vi "GlueRepeatedLinePattern-TeachMode.vi"(0 "Calibration Directory":path, 1 "Module Number":i32=7, 2 "Stereo Angle [mrad]":dbl=-26.0 format="%#_13g", 3 "Dry Run":bool, 4 "Controller In":refnum<k24>) -> ()   [LabVIEW 2016]
uses:
  <vilib>/LabVIEW Interface for Arduino/Type Defs/Arduino Resource.ctl
  <vilib>/LabVIEW Interface for Arduino/Type Defs/Board Type.ctl
  C:/Users/Aerotech/Documents/BNLStaveAssembly-blueprint/Bin/Aerotech.A3200.dll
  BNLStaveAssembly-blueprint/Bin/Aerotech.A3200.dll
  <vilib>/LabVIEW Interface for Arduino/Type Defs/Pin Mode.ctl
  <vilib>/Utility/file.llb/Read Delimited Spreadsheet (DBL).vi
  <vilib>/LabVIEW Interface for Arduino/LabVIEW Interface for Arduino.lvlib
panel:
  out "N Lines":i32
  out "Lines Glued":i32
  out "Elapsed Time [s]":dbl format="%.2g"
  out "Finished":bool
  in  "Abort stage":bool
  in  "Pattern Indicator":enum32{"Glue Pattern"}(tab)
  out "Relative Line\nSeparations [mm]":dbl[][](array[numeric])=[[18.5, 7.25], [2.5, 3.5], [-3.5, 5.0], [2.5, 3.15], [2.5, 3.15], [2.5, 3.15], [2.5, 3.15], [2.5, 3.15], [2.5, 3.15], [2.5, 3.15], [2.5, 3.15], [2.5, 3.15], [2.5, 3.15], [2.5, 3.15], [3.75, 5.0], [2.5, 3.5]] format="%#_13g"
  out "Line Lengths [mm]":dbl[](array[numeric])=[65.0, 65.0, 73.5, 73.5, 73.5, 73.5, 73.5, 73.5, 73.5, 73.5, 73.5, 73.5, 73.5, 73.5, 65.0, 65.0] format="%#_13g"
  out "Line Speeds [mm/s]":dbl[][](array[numeric])=[[5.0, 5.0, 75.0, 75.0, 75.0, 75.0], [5.0, 5.0, 0.0, 0.0, 0.0, 0.0], [7.5, 7.5, 0.0, 0.0, 0.0, 0.0], [7.5, 7.5, 0.0, 0.0, 0.0, 0.0], [7.5, 7.5, 0.0, 0.0, 0.0, 0.0], [7.5, 7.5, 0.0, 0.0, 0.0, 0.0], [7.5, 7.5, 0.0, 0.0, 0.0, 0.0], [7.5, 7.5, 0.0, 0.0, 0.0, 0.0], [7.5, 7.5, 0.0, 0.0, 0.0, 0.0], [7.5, 7.5, 0.0, 0.0, 0.0, 0.0], [7.5, 7.5, 0.0, 0.0, 0.0, 0.0], [7.5, 7.5, 0.0, 0.0, 0.0, 0.0], [7.5, 7.5, 0.0, 0.0, 0.0, 0.0], [7.5, 7.5, 0.0, 0.0, 0.0, 0.0], [5.0, 5.0, 0.0, 0.0, 0.0, 0.0], [5.0, 5.0, 0.0, 0.0, 0.0, 0.0]] format="%#_13g"
  in  "Outputs Tab":enum32{"Running Positions"}(tab)
  out "Running Positions [mm]":dbl[][](array[numeric])
  in  "Times [s]":dbl[](array[numeric])
  out "Running Times [s]":dbl[](array[numeric])
  in  "Inputs Tab":T1(tab)
  out "Virtual Stave Map":path
  out "Stave Angle [rad]":dbl format="%#_13g"
  out "Total Angle [rad]":dbl
  in  "Pause Before Line [ms]":dbl=500.0 format="%#_13g"
  out "Arduino Resource":T2={"VISA resource"="GlueCTRL", "Board Type"=enum."Uno", "Connection Type"=enum."USB / Serial", "Bytes Per Packet (15)"=15}
  in  "Digital I/O Pin":u8=7
  in  "Default Axis Speeds":T4={"X [mm/s]"=25.0, "Y [mm/s]"=25.0, "Z [mm/s]"=25.0}
  in  "Pause After Line [ms]":dbl=1000.0 format="%#_13g"
  in  "Fine Axis Speeds [mm/s]":T4={"X [mm/s]"=15.0, "Y [mm/s]"=15.0, "Z [mm/s]"=15.0}
  in  "Camera to Dispenser Shift [mm]":dbl[](array[numeric])=[100.0, 0.0, -10.0]
  in  "Glue Pattern .csv File":path=path "C:/Users/Aerotech/Documents/BNL_ThermomechanicalStave/SchillaciGlue/GluePatterns/TimingAccuracy.txt"
  in  "Axial":bool
  in  "Positions [mm]":dbl[][](array[numeric])
  in  "Terminate":bool
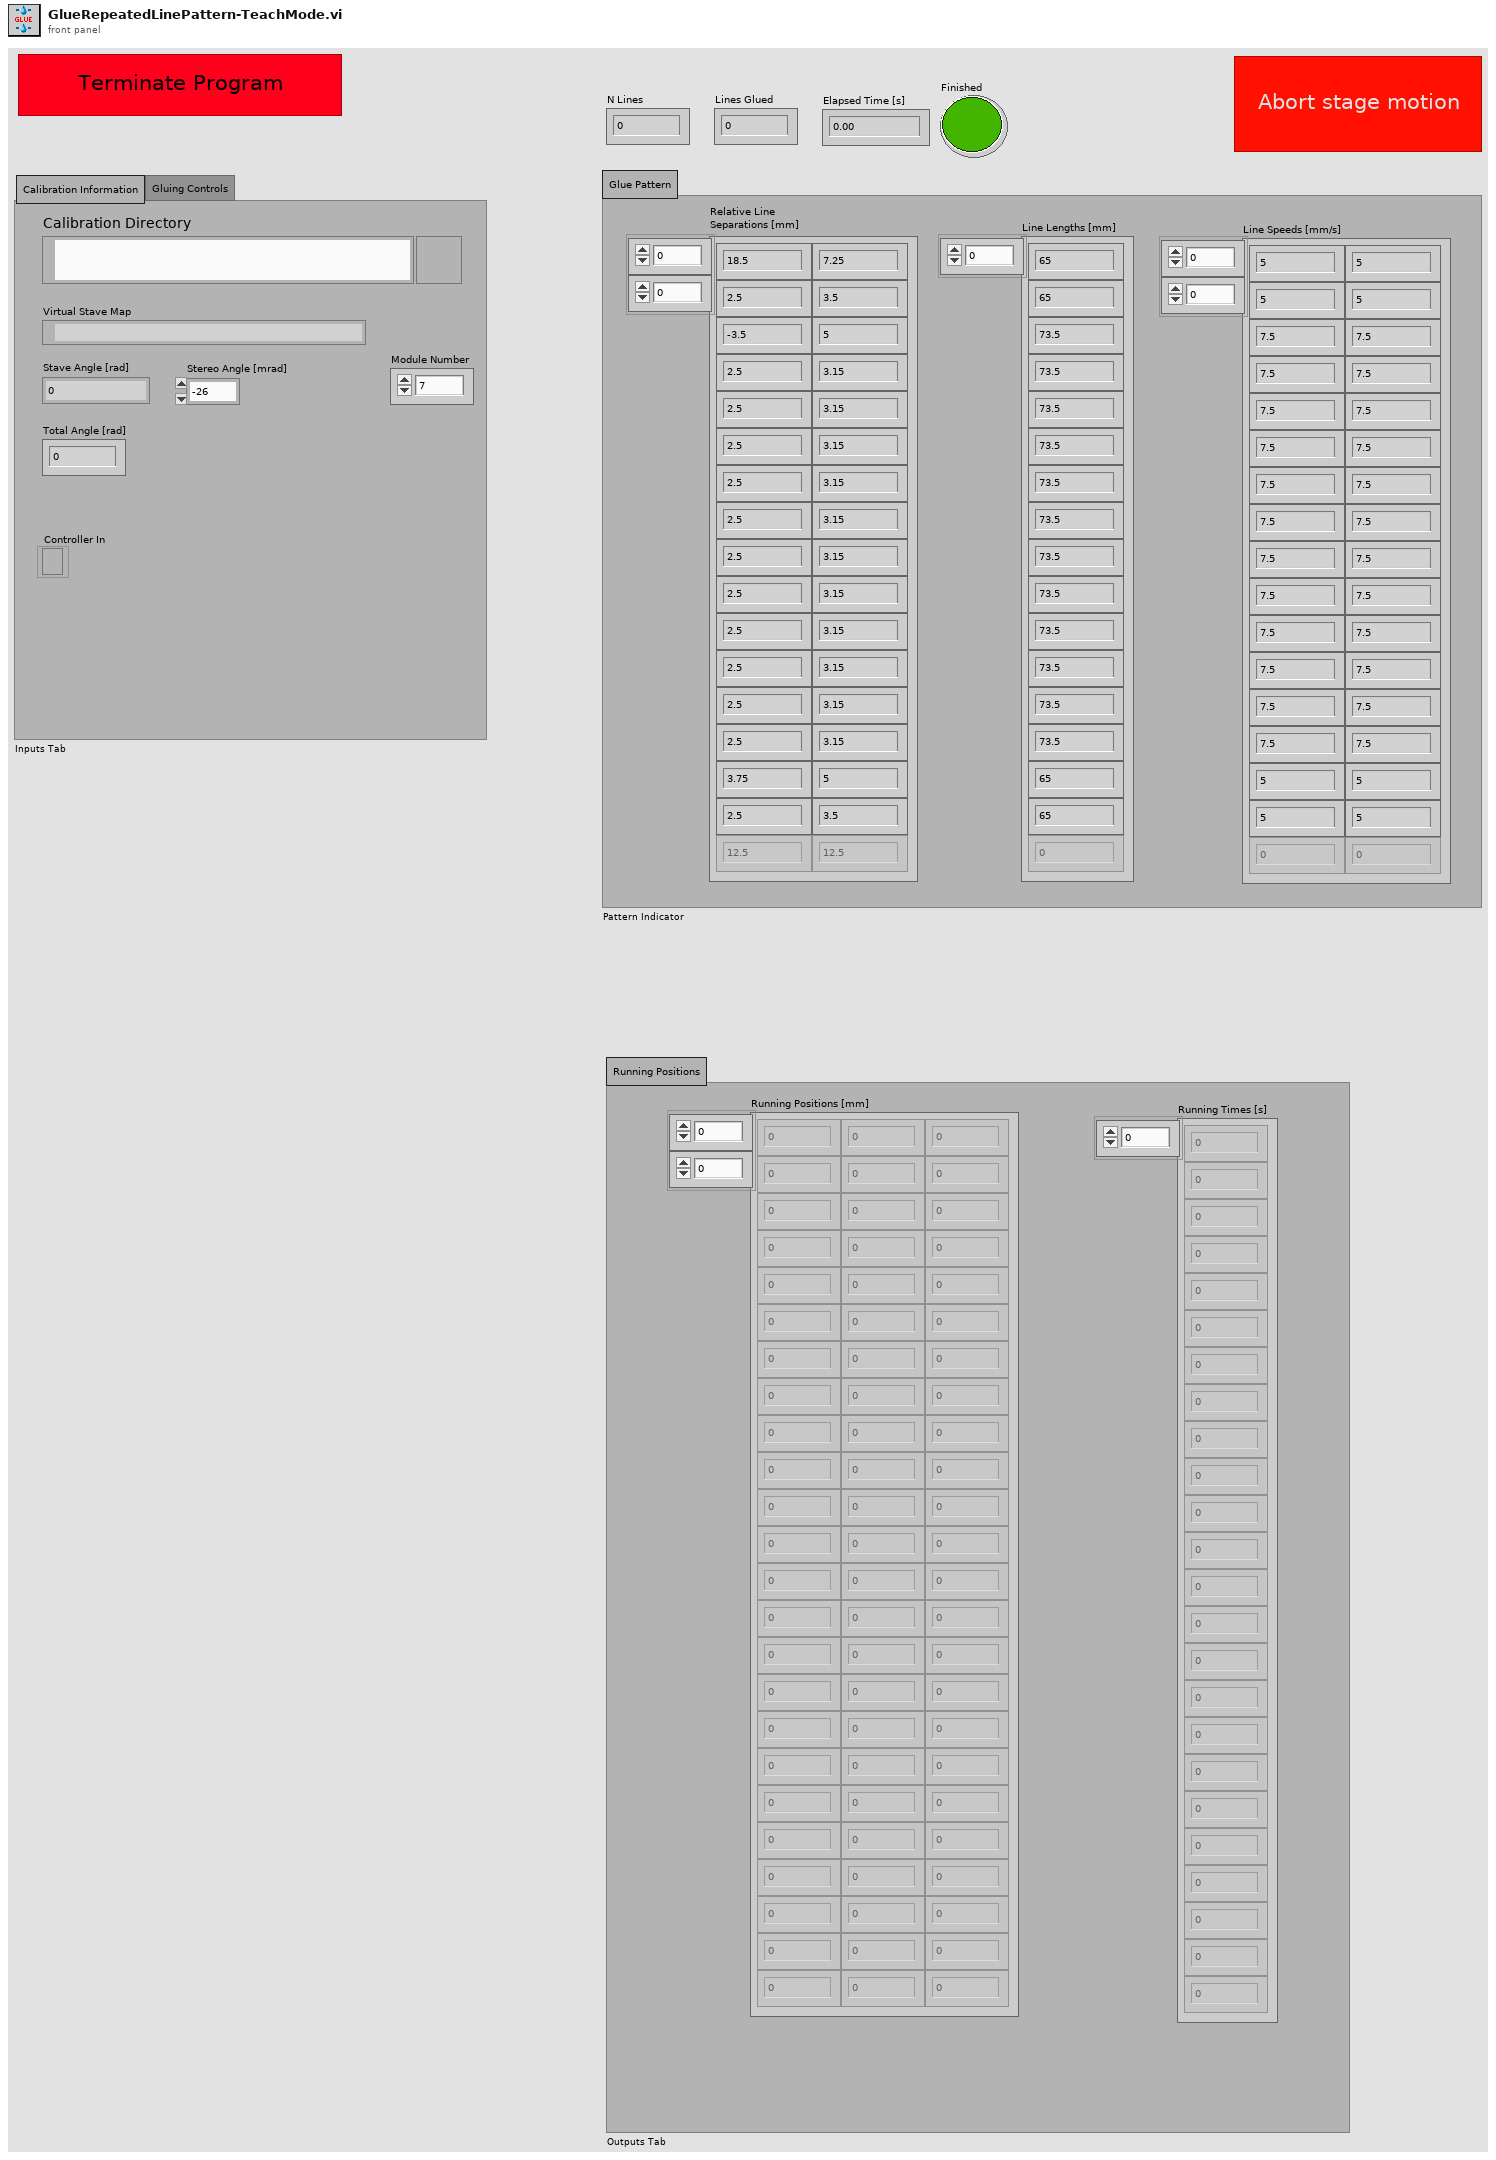
[diagram p1: front panel]
types:
  T1 = enum32{"Calibration Information", "Gluing Controls"}
  T2 = typedef "LabVIEW Interface for Arduino.lvlib/Arduino Resource.ctl" = cluster{"VISA resource":refnum<visa-resource-name>, "Board Type":T3, "Connection Type":enum8{"USB / Serial"}, "Bytes Per Packet (15)":u8}
  T3 = typedef "LabVIEW Interface for Arduino.lvlib/Board Type.ctl" = enum16{"Uno", "Dimuelanove w/Atmega 328", "Mega 2560"}
  T4 = cluster{"X [mm/s]":dbl, "Y [mm/s]":dbl, "Z [mm/s]":dbl}
  T5 = typedef "LabVIEW Interface for Arduino.lvlib/Pin Mode.ctl" = enum8{"Input", "Output"}
  T6 = cluster{"Final X":dbl, "Final Y":dbl, "Final Z":dbl}
  T7 = cluster{"Numeric":dbl, "Numeric":dbl, "Z [mm/s]":dbl}
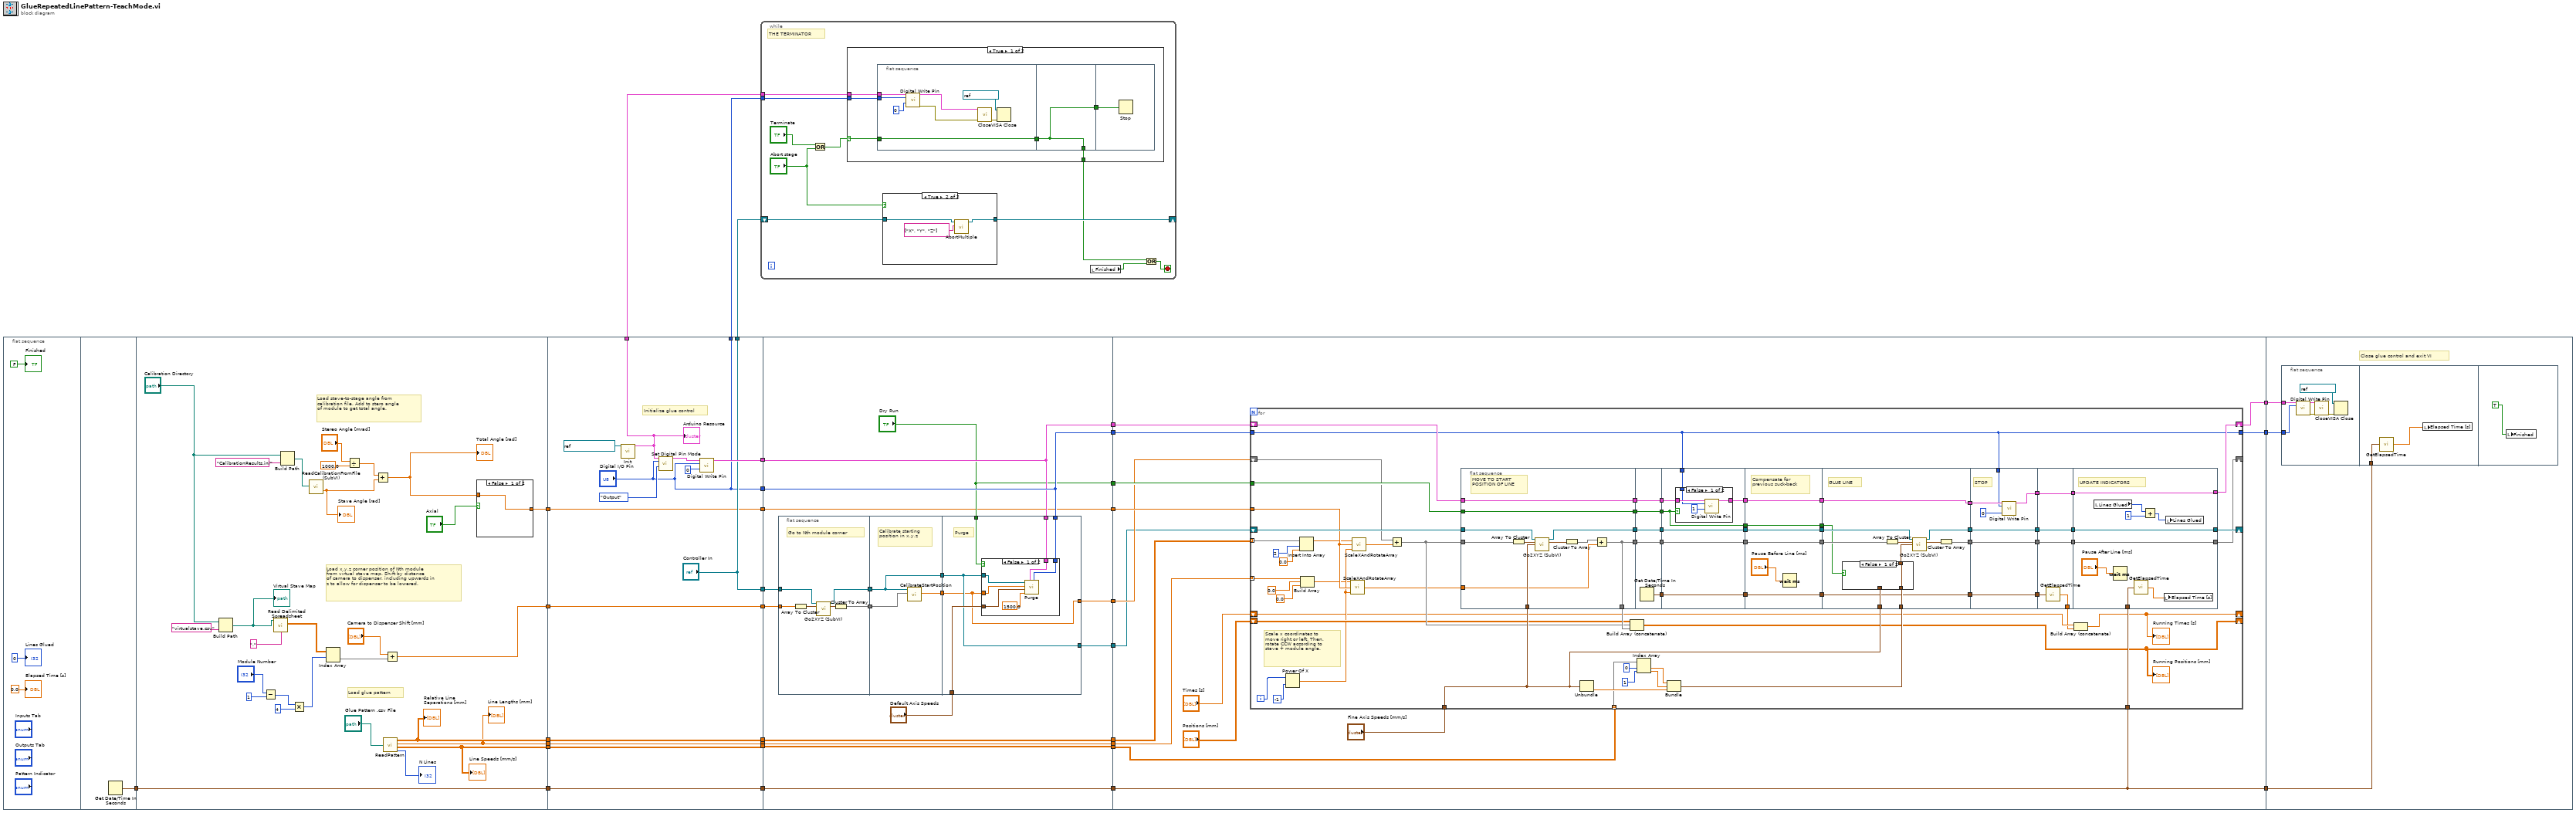
[diagram p0: block diagram]
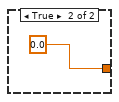
[diagram p2: hidden frame]
diagram:
  n1 = flat-sequence {
    tunnel: [w36] -> w16
    tunnel: [w49] -> w32
    tunnel: w16 -> [w46]
    tunnel: [w46] -> w15
    tunnel: [w38] -> w11
    tunnel: [w42] -> w5
    tunnel: [w41] -> w4
    tunnel: [w40] -> w2
    tunnel: w32 -> [w76]
    tunnel: [w76] -> w31
    tunnel: ["Controller In"] -> w30
    tunnel: [w75] -> w29
    tunnel: ["Digital I/O Pin"] -> w28
    tunnel: [w74] -> w22
    tunnel: ["Controller In"] -> w21
    tunnel: [w71] -> w18
    tunnel: w15 -> [w72]
    tunnel: [w72] -> w14
    tunnel: w11 -> [w71]
    tunnel: ["Digital I/O Pin"] -> w10
    tunnel: [w69] -> w6
    tunnel: w5 -> [w69]
    tunnel: w4 -> [w68]
    tunnel: [w68] -> w3
    tunnel: w2 -> [w67]
    tunnel: [w67] -> w1
    tunnel: w31 -> [w92]
    tunnel: w30 -> [w91]
    tunnel: w29 -> [w89]
    tunnel: w28 -> [w90]
    tunnel: [w90] -> w25
    tunnel: [w89] -> w24
    tunnel: [w88] -> w23
    tunnel: ["Dry Run"] -> w20
    tunnel: [w86] -> w19
    tunnel: w18 -> [w86]
    tunnel: [w85] -> w17
    tunnel: w14 -> [w84]
    tunnel: [w84] -> w13
    tunnel: [w83] -> w9
    tunnel: [w82] -> w8
    tunnel: [w81] -> w7
    tunnel: w6 -> [w83]
    tunnel: w3 -> [w82]
    tunnel: w1 -> [w81]
    tunnel: [w120] -> w27
    tunnel: [w131] -> w26
    tunnel: w25 -> [w130]
    tunnel: w24 -> [w129]
    tunnel: w23 -> [w125]
    tunnel: w20 -> [w128]
    tunnel: w19 -> [w127]
    tunnel: w17 -> [w126]
    tunnel: w13 -> [w124]
    tunnel: [w124] -> w12
    tunnel: w9 -> [w123]
    tunnel: w8 -> [w121]
    tunnel: w7 -> [w122]
    tunnel: w27 -> [w273]
    tunnel: w26 -> [w272]
    tunnel: w12 -> [w271]
    frame #0 {
      "Finished" <- FALSE ("Finished")
      "Elapsed Time [s]" <- 0.0 ("Elapsed Time [s]")
      "Lines Glued" <- 0 ("N Lines")
    }
    frame #1 {
      n2 = Get Date/Time In Seconds() -> (seconds since 1Jan1904=w36:timestamp)
    }
    frame #2 {
      # "Load glue pattern"
      # "Load x,y,z corner position of Nth module\nfrom virtual stave map. Shift by distance\nof camera to dispenser, including upwards in\nz to allow for dispenser to be lowered."
      # "Load stave-to-stage angle from\ncalibration file. Add to stero angle\nof module to get total angle."
      n3 = Build Path(base path="Calibration Directory", name or relative path="virtualstave.csv") -> (appended path=w58:path)
      "Virtual Stave Map" <- w58
      n4 = Subtract(x="Module Number", y=1) -> (x-y=w54:i32)
      n5 = call-poly <vilib>:"Read Delimited Spreadsheet.vi"("file path (dialog if empty)"=w58, "delimiter (\\t)"="," ("delimiter (\\t)")) -> ("all rows"=w50:dbl[][])  [unwired: 8 in, 5 out]
      n6 = Build Path(base path="Calibration Directory", name or relative path="CalibrationResults.ini") -> (appended path=w60:path)
      n7 = Multiply(x=w54, y=4) -> (x*y=w47:i32)
      n8 = call "ReadCalibrationFromFile (SubVI).vi"("Calibration file path"=w60) -> ("Angle"=w51:dbl)  [unwired: 12 in, 6 out]
      "Stave Angle [rad]" <- w51
      n9 = Index Array(array=w50, index (row)=w47) -> (element=w48:dbl[])  [unwired: 1 in]
      n10 = Divide(x="Stereo Angle [mrad]", y=1000.0) -> (x/y=w52:dbl)
      n11 = Add(x=w52, y=w51) -> (x+y=w37:dbl)
      "Total Angle [rad]" <- w37
      n12 = call "ReadPattern.vi"("file path (dialog if empty)"="Glue Pattern .csv File") -> ("Relative Line\nSeparations [mm]"=w42:dbl[][], "Line Lengths [mm]"=w41:dbl[], "Line Speeds [mm/s]"=w40:dbl[][], "N Lines"=→"N Lines":i32)
      "Relative Line\nSeparations [mm]" <- w42
      "Line Lengths [mm]" <- w41
      "Line Speeds [mm/s]" <- w40
      n13 = Add(x="Camera to Dispenser Shift [mm]", y=w48) -> (x+y=w49:dbl[])
      n14 = case shown="False" "Axial" {
        tunnel: [w65 0.0] -> w38
        tunnel: w37 -> [w65 _]
        frame False {
        }
        frame True {
        }
      }
    }
    frame #3 {
      # "Initialize glue control"
      n15 = call <vilib>:"Init.vi"("VISA resource"=refnum<visa-resource-name> "GlueCTRL") -> ("Arduino Resource"=w74:T2)  [unwired: 17 in, 1 out]
      "Arduino Resource" <- w74
      n16 = call <vilib>:"Set Digital Pin Mode.vi"("Arduino Resource"=w74, "Digital I/O Pin"="Digital I/O Pin", "Pin Mode (Input)"=Pin_Mode."Output") -> ("Arduino Resource"=w78:T2)  [unwired: 11 in, 1 out]
      n17 = call <vilib>:"Digital Write Pin.vi"("Arduino Resource"=w78, "Digital I/O Pin (0)"="Digital I/O Pin", "Value (0)"=u8 0) -> ("Arduino Resource"=w75:T2)  [unwired: 11 in, 1 out]
    }
    frame #4 {
      n18 = flat-sequence {
        tunnel: w91 -> [w101]
        tunnel: [w100] -> w97
        tunnel: w92 -> [w99]
        tunnel: [w98] -> w96
        tunnel: w97 -> [w105]
        tunnel: w96 -> [w106]
        tunnel: [w105] -> w95
        tunnel: [w104] -> w94
        tunnel: w95 -> [w109]
        tunnel: w94 -> [w107]
        tunnel: "Default Axis Speeds" -> [w112]
        tunnel: w90 -> [w111]
        tunnel: w89 -> [w110]
        tunnel: [w109] -> w88
        tunnel: "Dry Run" -> [w108]
        tunnel: [w107] -> w85
        frame #0 {
          # "Go to Nth module corner"
          n19 = Array To Cluster(array=w99) -> (cluster=w103:cluster{"[0]":dbl, "[1]":dbl, "[2]":dbl})
          n20 = call "Go2XYZ (SubVI).vi"(".NET Refnum in"=w101, "Go to Coordinates"=w103) -> (".NET Refnum out"=w100:refnum<k24>, "Final Position"=w102:T6)  [unwired: 9 in, 3 out]
          n21 = Cluster To Array(cluster=w102) -> (array=w98:dbl[])
        }
        frame #1 {
          # "Calibrate starting\nposition in x,y,z"
          n22 = call "CalibrateStartPosition.vi"("Start Position [mm]"=w106, ".NET Refnum In"=w105) -> ("Final Position [mm]"=w104:dbl[])  [unwired: 9 in]
        }
        frame #2 {
          # "Purge"
          n23 = case shown="False" w108 {
            tunnel: w112 -> [w115 _]
            tunnel: w111 -> [w118 _]
            tunnel: w110 -> [w117 _]
            tunnel: w109 -> [w113 _]
            tunnel: w107 -> [w114 _]
            frame False {
              n24 = call "Purge.vi"("Digital I/O Pin"=w118, "Arduino Resource"=w117, "Purge Time [ms]"=1500.0, "Axis Speeds"=w115, "Start Position [mm]"=w114, ".NET Refnum In"=w113) -> ()  [unwired: 6 in]
            }
            frame True {
            }
          }
        }
      }
    }
    frame #5 {
      n25 = for {
        tunnel: w123 -> [w197] mode=indexing
        tunnel: w121 -> [w198] mode=indexing
        shift-right: [w175] -> _
        shift-left: w126 -> [w170]
        tunnel: w122 -> [w179] mode=indexing
        shift-right: [w177] -> _
        shift-left: w125 -> [w184]
        shift-right: [w188] -> w120
        shift-left: w129 -> [w182]
        shift-right: [w134] -> _
        shift-left: "Positions [mm]" -> [w178]
        tunnel: w130 -> [w146]
        tunnel: [w146] -> w131
        tunnel: "Fine Axis Speeds [mm/s]" -> [w183]
        tunnel: w128 -> [w181]
        tunnel: w127 -> [w174]
        tunnel: w124 -> [w171]
        shift-right: [w135] -> _
        shift-left: "Times [s]" -> [w153]
        i -> [w172]
        # "Scale x coordinates to\nmove right or left. Then,\nrotate CCW according to\nstave + module angle."
        n26 = Power Of X(1:-1 ("x"), 2:w172) -> (0:w173:dbl)
        n27 = Insert Into Array(array=w197, index=2, new element=0.0 ("new element/subarray")) -> (w169:dbl[])
        n28 = Build Array(w198, 0.0 ("element"), 0.0 ("element")) -> (w167:dbl[])
        n29 = call "ScaleXAndRotateArray.vi"("Scale"=w173, "Angle"=w174, "X, Y, Z Input"=w167) -> ("c * X', Y', Z Output"=w166:dbl[])
        n30 = call "ScaleXAndRotateArray.vi"("Scale"=w173, "Angle"=w174, "X, Y, Z Input"=w169) -> ("c * X', Y', Z Output"=w168:dbl[])
        n31 = Add(x=w170, y=w168) -> (x+y=w180:dbl[])
        n32 = flat-sequence {
          tunnel: w181 -> [w211]
          tunnel: w184 -> [w207]
          tunnel: w182 -> [w212]
          tunnel: [w212] -> w165
          tunnel: [w206] -> w164
          tunnel: [w210] -> w163
          tunnel: [w211] -> w162
          tunnel: [w210] -> w185
          tunnel: w183 -> [w205]
          tunnel: w180 -> [w203]
          tunnel: w166 -> [w202]
          tunnel: w165 -> [w217]
          tunnel: [w217] -> w151
          tunnel: w164 -> [w216]
          tunnel: [w216] -> w150
          tunnel: w163 -> [w215]
          tunnel: [w215] -> w149
          tunnel: w162 -> [w214]
          tunnel: [w214] -> w148
          tunnel: [w213] -> w147
          tunnel: w151 -> [w220]
          tunnel: w150 -> [w224]
          tunnel: [w224] -> w145
          tunnel: w149 -> [w223]
          tunnel: [w223] -> w143
          tunnel: w148 -> [w218]
          tunnel: [w218] -> w141
          tunnel: w147 -> [w222]
          tunnel: [w222] -> w139
          tunnel: w146 -> [w221]
          tunnel: [w219] -> w137
          tunnel: w145 -> [w235]
          tunnel: [w235] -> w144
          tunnel: w143 -> [w234]
          tunnel: [w234] -> w142
          tunnel: w141 -> [w233]
          tunnel: [w233] -> w140
          tunnel: w139 -> [w232]
          tunnel: [w232] -> w138
          tunnel: w137 -> [w231]
          tunnel: [w231] -> w136
          tunnel: w194 -> [w241]
          tunnel: [w236] -> w189
          tunnel: [w240] -> w186
          tunnel: w144 -> [w244]
          tunnel: w142 -> [w246]
          tunnel: w140 -> [w243]
          tunnel: w183 -> [w239]
          tunnel: [w238] -> w176
          tunnel: [w237] -> w154
          tunnel: w138 -> [w237]
          tunnel: w136 -> [w236]
          tunnel: w189 -> [w256]
          tunnel: w146 -> [w254]
          tunnel: [w255] -> w161
          tunnel: w186 -> [w252]
          tunnel: [w252] -> w159
          tunnel: [w251] -> w157
          tunnel: w176 -> [w251]
          tunnel: [w250] -> w155
          tunnel: w154 -> [w250]
          tunnel: w161 -> [w261]
          tunnel: [w261] -> w160
          tunnel: w159 -> [w260]
          tunnel: [w260] -> w158
          tunnel: w157 -> [w259]
          tunnel: [w259] -> w156
          tunnel: w155 -> [w258]
          tunnel: [w257] -> w152
          tunnel: [w270] -> w188
          tunnel: w160 -> [w270]
          tunnel: [w269] -> w177
          tunnel: w158 -> [w269]
          tunnel: [w268] -> w175
          tunnel: w156 -> [w268]
          tunnel: w171 -> [w264]
          frame #0 {
            # "MOVE TO START\nPOSITION OF LINE"
            n33 = Array To Cluster(array=w203) -> (cluster=w204:cluster{"[0]":dbl, "[1]":dbl, "[2]":dbl})
            n34 = call "Go2XYZ (SubVI).vi"(".NET Refnum in"=w207, "Go to Coordinates"=w204, "Axis Speeds"=w205) -> (".NET Refnum out"=w206:refnum<k24>, "Final Position"=w208:T6)  [unwired: 8 in, 3 out]
            n35 = Cluster To Array(cluster=w208) -> (array=w209:dbl[])
            n36 = Add(x=w209, y=w202) -> (x+y=w210:dbl[])
          }
          frame #1 {
            n37 = Get Date/Time In Seconds() -> (seconds since 1Jan1904=w213:timestamp)
          }
          frame #2 {
            n38 = case shown="False" w218 {
              tunnel: [w228 w229] -> w219
              tunnel: w220 -> [w227 w229]
              tunnel: w221 -> [w226 _]
              frame False {
                n39 = call <vilib>:"Digital Write Pin.vi"("Arduino Resource"=w227, "Digital I/O Pin (0)"=w226, "Value (0)"=u8 1) -> ("Arduino Resource"=w228:T2)  [unwired: 11 in, 1 out]
              }
              frame True {
              }
            }
          }
          frame #3 {
            # "Compensate for\nprevious suck-back"
            n40 = Wait (ms)(milliseconds to wait="Pause Before Line [ms]") -> ()  [unwired: 1 out]
          }
          frame #4 {
            # "GLUE LINE"
            n41 = case shown="False" w243 {
              tunnel: [w248 w249] -> w242
              tunnel: w241 -> [w248 _]
              tunnel: w239 -> [_ w249]
              frame False {
              }
              frame True {
              }
            }
            n42 = Array To Cluster(array=w246) -> (cluster=w245:cluster{"[0]":dbl, "[1]":dbl, "[2]":dbl})
            n43 = call "Go2XYZ (SubVI).vi"(".NET Refnum in"=w244, "Go to Coordinates"=w245, "Axis Speeds"=w242) -> (".NET Refnum out"=w240:refnum<k24>, "Final Position"=w247:T6)  [unwired: 8 in, 3 out]
            n44 = Cluster To Array(cluster=w247) -> (array=w238:dbl[])
          }
          frame #5 {
            # "STOP"
            n45 = call <vilib>:"Digital Write Pin.vi"("Arduino Resource"=w256, "Digital I/O Pin (0)"=w254, "Value (0)"=u8 0) -> ("Arduino Resource"=w255:T2)  [unwired: 11 in, 1 out]
          }
          frame #6 {
            n46 = call "GetElapsedTime.vi"("Start Time"=w258) -> ("Elapsed Time [s]"=w257:sgl)
          }
          frame #7 {
            # "UPDATE INDICATORS"
            n47 = local read "Lines Glued"() -> (w266:i32)
            n48 = Wait (ms)(milliseconds to wait="Pause After Line [ms]") -> ()  [unwired: 1 out]
            n49 = call "GetElapsedTime.vi"("Start Time"=w264) -> ("Elapsed Time [s]"=w263:sgl)
            n50 = Add(x=w266, y=1) -> (x+y=w267:i32)
            n51 = local write "Elapsed Time [s]"(w263) -> ()
            n52 = local write "Lines Glued"(w267) -> ()
          }
        }
        n53 = Unbundle(w183) -> ("Z [mm/s]"=w187:dbl)  [unwired: 2 out]
        n54 = Build Array (concatenate)(w178, w180, w185) -> (w134:dbl[][])
        "Running Positions [mm]" <- w134
        n55 = Index Array(array=w179, index #1=0 ("index"), index #2=1 ("index")) -> (element #1=w190:dbl, element #2=w191:dbl)
        n56 = Bundle("Numeric"=w190, "Numeric"=w191, "Z [mm/s]"=w187) -> (w194:T7)  [unwired: 1 in]
        n57 = Build Array (concatenate)(w153, w152) -> (w135:dbl[])
        "Running Times [s]" <- w135
      }
    }
    frame #6 {
      # "Close glue control and exit VI"
      n58 = flat-sequence {
        tunnel: w273 -> [w275]
        tunnel: w272 -> [w274]
        tunnel: w271 -> [w280]
        frame #0 {
          n59 = call <vilib>:"Digital Write Pin.vi"("Arduino Resource"=w275, "Digital I/O Pin (0)"=w274) -> ("Arduino Resource"=w278:T2, "error out"=w277:errorcluster)  [unwired: 12 in]
          n60 = call <vilib>:"Close.vi"("Arduino Resource"=w278, "error in"=w277) -> ("error out"=w276:errorcluster)  [unwired: 13 in]
          n61 = VISA Close(VISA resource name=refnum<visa-resource-name> "GlueCTRL", error in (no error)=w276) -> ()  [unwired: 1 out]
        }
        frame #1 {
          n62 = call "GetElapsedTime.vi"("Start Time"=w280) -> ("Elapsed Time [s]"=w281:sgl)
          n63 = local write "Elapsed Time [s]"(w281) -> ()
        }
        frame #2 {
          n64 = local write "Finished"(TRUE ("stop? (T)")) -> ()
        }
      }
    }
  }
  n65 = while {
    tunnel: w22 -> [w292]
    shift-right: [w290] -> _
    shift-left: w21 -> [w291]
    tunnel: w10 -> [w284]
    stop <- w287 stop-if-true
    # "THE TERMINATOR"
    n66 = Or(x="Terminate", y="Abort stage") -> (x .or. y?=w286:bool)
    n67 = case shown="True" w286 {
      selector: w286 -> [w302 w313]
      tunnel: w292 -> [w300 _]
      tunnel: [w298 w313] -> w285
      tunnel: w284 -> [w297 _]
      frame True {
        n68 = flat-sequence {
          tunnel: [w308] -> w301
          tunnel: w297 -> [w304]
          tunnel: w300 -> [w306]
          tunnel: w302 -> [w308]
          tunnel: w301 -> [w311]
          tunnel: [w311] -> w299
          tunnel: [w311] -> w298
          tunnel: w299 -> [w312]
          frame #0 {
            n69 = call <vilib>:"Digital Write Pin.vi"("Arduino Resource"=w306, "Digital I/O Pin (0)"=w304, "Value (0)"=u8 0) -> ("Arduino Resource"=w307:T2, "error out"=w303:errorcluster)  [unwired: 11 in]
            n70 = call <vilib>:"Close.vi"("Arduino Resource"=w307, "error in"=w303) -> ("error out"=w309:errorcluster)  [unwired: 13 in]
            n71 = VISA Close(VISA resource name=refnum<visa-resource-name> "GlueCTRL", error in (no error)=w309) -> ()  [unwired: 1 out]
          }
          frame #1 {
          }
          frame #2 {
            n72 = Stop(stop? (T)=w312) -> ()
          }
        }
      }
      frame False {
      }
    }
    n73 = case shown="True" "Abort stage" {
      tunnel: w291 -> [w293 w295]
      tunnel: [w293 w294] -> w290
      frame False {
      }
      frame True {
        n74 = call "AbortMultiple.vi"("axis names"=string[] ["X", "Y", "Z"], "controller in"=w295) -> ("controller out"=w294:refnum<k24>)  [unwired: 8 in, 1 out]
      }
    }
    n75 = local read "Finished"() -> (w283:bool)
    n76 = Or(x=w285, y=w283) -> (x .or. y?=w287:bool)
  }
